vi "GetInfo.vi"(8 "Error In":errorcluster, 11 "reference in":refnum<class "Rectangle.lvclass">) -> (0 "Error Out":errorcluster, 2 "Console":string, 3 "reference out":refnum<class "Rectangle.lvclass">)   [LabVIEW 2020, in "Rectangle.lvclass"]
uses:
  Rectangle.lvclass
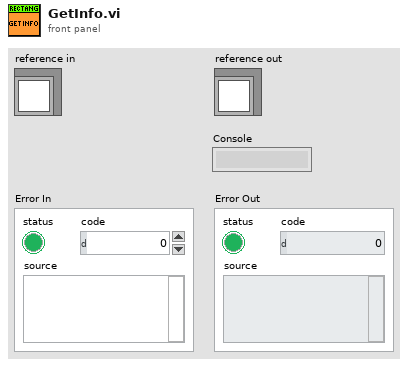
[diagram p1: front panel]
types:
  T1 = typedef "Rectangle.lvclass/ObjectAttributes.ctl" = cluster{"_width":i32, "_height":i32}
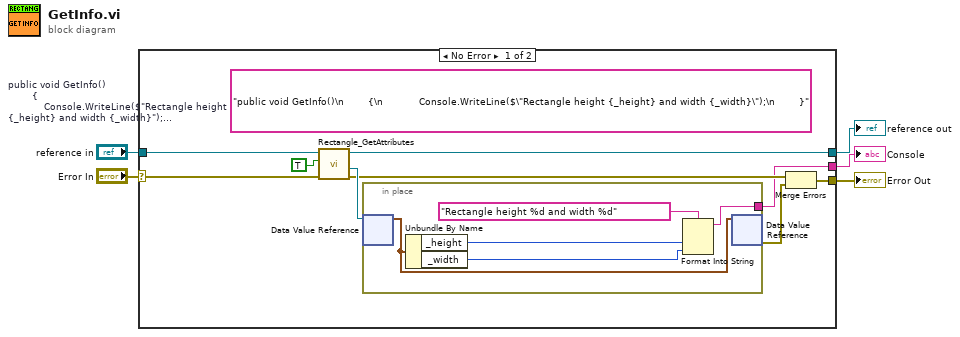
[diagram p0: block diagram]
diagram:
  n1 = case shown="No Error" "Error In" {
    selector: "Error In" -> [w13 w21]
    tunnel: [w10 w21] -> w4
    tunnel: [w11 w20] -> w2
    tunnel: "reference in" -> [w14 w20]
    tunnel: [w6 _] -> w1
    frame No Error {
      (unwired) "public void GetInfo()\n        {\n            Console.WriteLine($\"Rectangle height {_height} and width {_width}\");\n        }"  # public void GetInfo()         {             Console.WriteLine($"Rectangle height {_height} and width {_width}");         }
      n2 = call "Rectangle_GetAttributes.vi"("error in (no error)"=w13, "OnlyGetDvrReference(False)"=TRUE, "reference in"=w14) -> ("error out"=w8:errorcluster, "DataRef"=w9:refnum<data-value>, "reference out"=w11:refnum<class "Rectangle.lvclass">)  [unwired: 5 in, 1 out]
      n3 = in-place {
        in-place-border: [w15] -> w6
        n4 = in-place-dvr #1(w9) -> (w16:T1)  [unwired: 1 out]
        n5 = Unbundle By Name(w16) -> ("_height"=w19:i32, "_width"=w18:i32)
        n6 = Format Into String(format string="Rectangle height %d and width %d", w19, w18) -> (resulting string=w15:string)  [unwired: 2 in, 1 out]
        n7 = in-place-dvr #1(w16) -> (w12:errorcluster)  [unwired: 1 out]
      }
      n8 = Merge Errors(w8, w12) -> (w10:errorcluster)
    }
    frame Error {
    }
  }
  "Error Out" <- w4
  "reference out" <- w2
  "Console" <- w1
